vi "ReversePointOrder.vi"(2 "error in (no error)":errorcluster, 3 "Points In (pixels)":dbl[][](array[numeric])) -> (0 "error out":errorcluster, 1 "Points Out (pixels) reversed":dbl[][](array[numeric]))   [LabVIEW 2010]
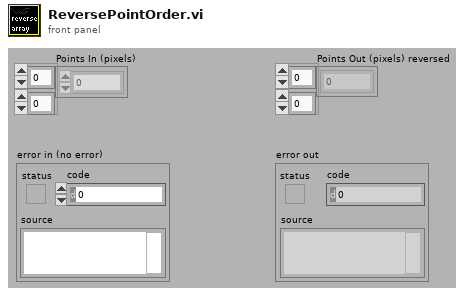
[diagram p1: front panel]
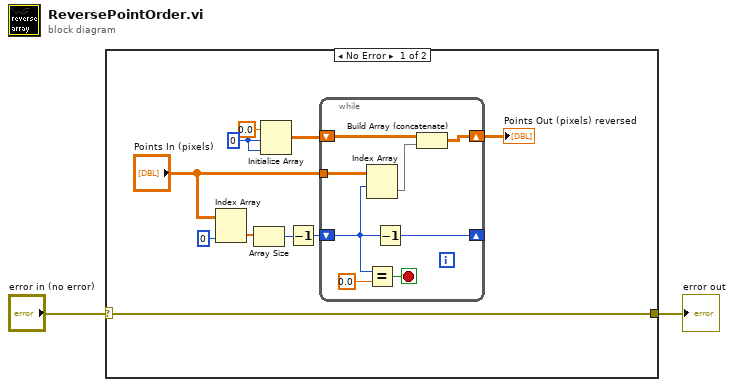
[diagram p0: block diagram]
diagram:
  n1 = case shown="No Error" "error in (no error)" {
    selector: "error in (no error)" -> [w7 w21]
    tunnel: [w7 w21] -> w1
    frame No Error {
      w6 = 0 ("dimension size")
      n2 = Index Array(array="Points In (pixels)", index (col)=0 ("disabled index (col)")) -> (element=w11:dbl[])  [unwired: 1 in]
      n3 = Array Size(array=w11) -> (size(s)=w4:i32)
      n4 = Initialize Array(0.0 ("element"), w6, w6) -> (w5:dbl[][])
      n5 = Decrement(x=w4) -> (x-1=w3:i32)
      n6 = while {
        shift-right: [w14] -> _
        shift-left: w3 -> [w13]
        shift-right: [w17] -> w8
        shift-left: w5 -> [w18]
        tunnel: "Points In (pixels)" -> [w20]
        stop <- w15 stop-if-true
        n7 = Index Array(array=w20, index (row)=w13) -> (element=w19:dbl[])  [unwired: 1 in]
        n8 = Equal?(x=w13, y=0.0) -> (x = y?=w15:bool)
        n9 = Decrement(x=w13) -> (x-1=w14:i32)
        n10 = Build Array (concatenate)(w18, w19) -> (w17:dbl[][])
      }
      "Points Out (pixels) reversed" <- w8
    }
    frame Error {
    }
  }
  "error out" <- w1
